vi "reconstrCluster.vi"() -> ()   [LabVIEW 2011]
panel:
  in  "clusterIndex (stop) 2":i32[](array[numeric])=[21, 21, 17, 13, 9]
  in  "clusterIndex":i32[](array[numeric])=[0, 5, 5, 10, 15, 20]
  in  "Cluster Names":string[](array[string])
  in  "Array 5":variant[](array[variant])
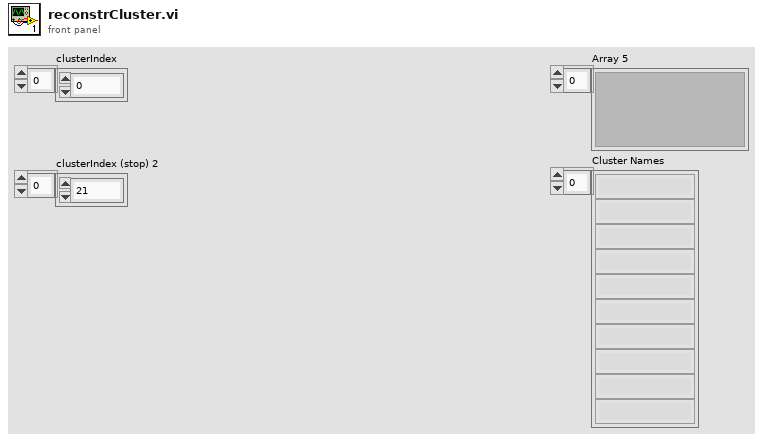
[diagram p1: front panel]
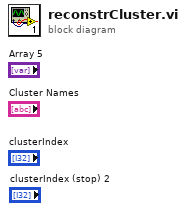
[diagram p0: block diagram]
diagram:
